vi "Read States.vi"(8 "error in (no error)":errorcluster, 11 "FollowAttackerTactic in":refnum<class "FollowAttackerTactic.lvclass">) -> (0 "error out":errorcluster, 2 "States":enum16{"Exit", "FollowAttacker"}(ring), 3 "FollowAttackerTactic out":refnum<class "FollowAttackerTactic.lvclass">)   [LabVIEW 2020, in "FollowAttackerTactic.lvclass"]
uses:
  FollowAttackerTactic.lvclass
  FollowAttackerTactic.lvclass/FollowAttackerTactic.ctl
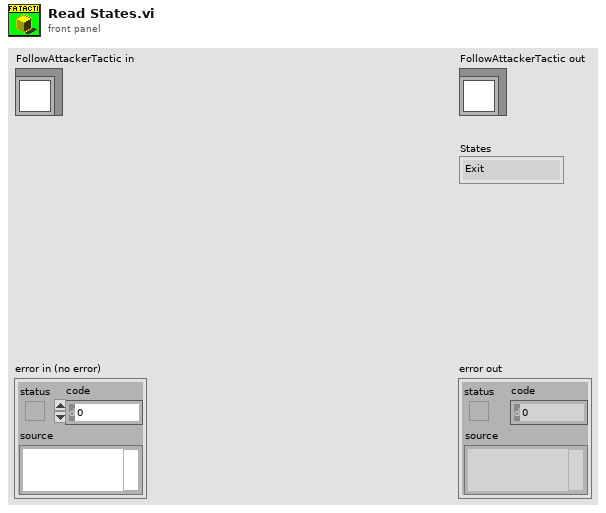
[diagram p1: front panel]
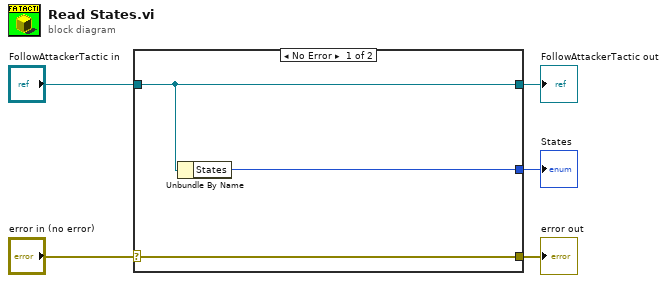
[diagram p0: block diagram]
diagram:
  n1 = case shown="No Error" "error in (no error)" {
    selector: "error in (no error)" -> [w8 w9]
    tunnel: [w8 w9] -> w4
    tunnel: [w7 w10] -> w2
    tunnel: "FollowAttackerTactic in" -> [w7 w10]
    tunnel: [w6 _] -> w1
    frame No Error {
      n2 = Unbundle By Name(w7) -> ("States"=w6:enum16{"Exit", "FollowAttacker"})
    }
    frame Error {
    }
  }
  "error out" <- w4
  "FollowAttackerTactic out" <- w2
  "States" <- w1
